vi "ParseTicNumber.vi"(5 "ReplyType [7-bit]":T1=enum."7-bit", 9 "Type":string(combo), 11 "Read":string) -> (2 "LSB                   MSB":bool[](array[boolean]) caption="Booleans", 3 "Value":i64)   [LabVIEW 2021]
uses:
  TicReplyStyle.ctl
panel:
  out "x-1":i32
  out "8bitBytes":bool[][](array[boolean])
  out "7bitBytes":bool[][](array[boolean])
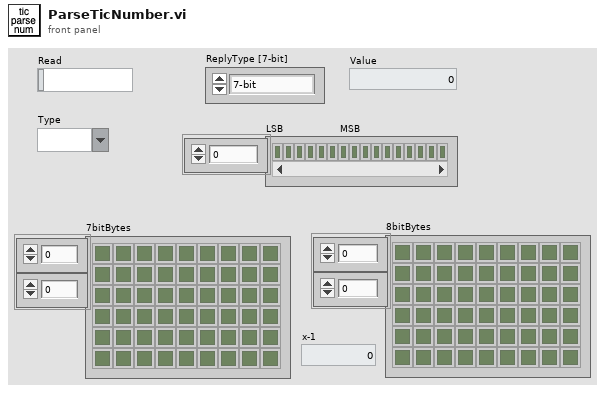
[diagram p1: front panel]
types:
  T1 = typedef "TicReplyStyle.ctl" = enum16{"8-bit", "7-bit"}
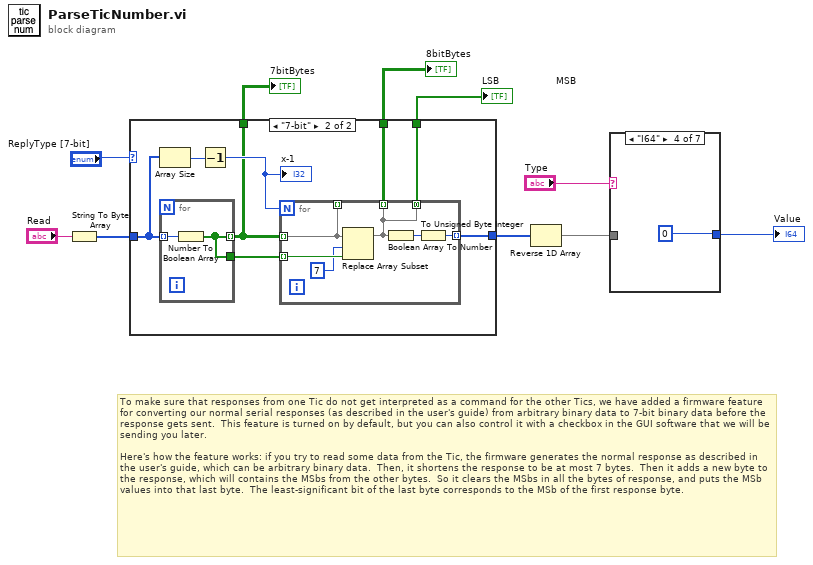
[diagram p0: block diagram]
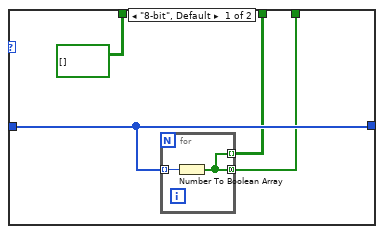
[diagram p2: hidden frame]
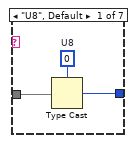
[diagram p3: hidden frame]
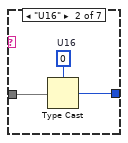
[diagram p4: hidden frame]
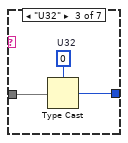
[diagram p5: hidden frame]
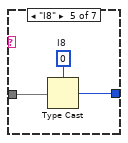
[diagram p6: hidden frame]
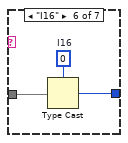
[diagram p7: hidden frame]
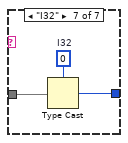
[diagram p8: hidden frame]
diagram:
  # "To make sure that responses from one Tic do not get interpreted as a command for the other Tics, we have added a firmware feature for converting our normal serial responses (as described in the user's guide) from arbitrary binary data to 7-bit binary data before the response gets sent.  This feature is turned on by default, but you can also control it with a checkbox in the GUI software that we will be sending you later.\n\nHere's how the feature works: if you try to read some data from the Tic, the firmware generates the normal response as described in the user's guide, which can be arbitrary binary data.  Then, it shortens the response to be at most 7 bytes.  Then it adds a new byte to the response, which will contains the MSbs from the other bytes.  So it clears the MSbs in all the bytes of response, and puts the MSb values into that last byte.  The least-significant bit of the last byte corresponds to the MSb of the first response byte."
  n1 = String To Byte Array(string="Read") -> (unsigned byte array=w8:u8[])
  n2 = case shown="\"7-bit\"" "ReplyType [7-bit]" {
    tunnel: w8 -> [w13 w19]
    tunnel: [w13 w23] -> w3
    tunnel: [bool[][] [] ("Boolean array") w22] -> w6
    tunnel: [w11 w21] -> w5
    tunnel: [w12 w18] -> w2
    frame "8-bit", Default {
      n3 = for {
        tunnel: w13 -> [w16] mode=indexing
        tunnel: [w15] -> w12 mode=concatenating
        tunnel: [w15] -> w11 mode=indexing
        n4 = Number To Boolean Array(number=w16) -> (Boolean array=w15:bool[])
      }
    }
    frame "7-bit" {
      n5 = Array Size(array=w19) -> (size(s)=w20:i32)
      n6 = for {
        tunnel: w19 -> [w32] mode=indexing
        tunnel: [w31] -> w22 mode=indexing
        tunnel: [w31] -> w17
        n7 = Number To Boolean Array(number=w32) -> (Boolean array=w31:bool[])
      }
      n8 = Decrement(x=w20) -> (x-1=w24:i32)
      "x-1" <- w24
      n9 = for {
        N: w24 -> [_]
        tunnel: w22 -> [w25] mode=indexing
        tunnel: w17 -> [w30] mode=indexing
        tunnel: [w27] -> w23 mode=indexing
        tunnel: [w26] -> w21 mode=indexing
        tunnel: [w26] -> w18 mode=concatenating
        tunnel: [w25] -> _ mode=indexing
        n10 = Replace Array Subset(array=w25, new element=w30, index=7) -> (w26:bool[])
        n11 = Boolean Array To Number(Boolean array=w26) -> (number=w28:u32)
        n12 = To Unsigned Byte Integer(number=w28) -> (unsigned 8bit integer=w27:u8)
      }
    }
  }
  "7bitBytes" <- w6
  "8bitBytes" <- w5
  "LSB                   MSB" <- w2
  n13 = Reverse 1D Array(array=w3) -> (reversed array=w1:u8[])
  n14 = case shown="\"I64\"" "Type" {
    tunnel: w1 -> [w34 w37 w40 _ w44 w47 w50]
    tunnel: [w33 w36 w39 i64 0 w43 w46 w49] -> w4
    frame "U8", Default {
      w35 = u8 0  # U8
      n15 = Type Cast(type=w35, x=w34) -> (*(type *) &x=w33:u8)
    }
    frame "U16" {
      w38 = u16 0  # U16
      n16 = Type Cast(type=w38, x=w37) -> (*(type *) &x=w36:u16)
    }
    frame "U32" {
      w41 = u32 0  # U32
      n17 = Type Cast(type=w41, x=w40) -> (*(type *) &x=w39:u32)
    }
    frame "I64" {
    }
    frame "I8" {
      w45 = i8 0  # I8
      n18 = Type Cast(type=w45, x=w44) -> (*(type *) &x=w43:i8)
    }
    frame "I16" {
      w48 = i16 0  # I16
      n19 = Type Cast(type=w48, x=w47) -> (*(type *) &x=w46:i16)
    }
    frame "I32" {
      w51 = 0  # I32
      n20 = Type Cast(type=w51, x=w50) -> (*(type *) &x=w49:i32)
    }
  }
  "Value" <- w4
